vi "RichToFlatnixnet_grpc_ConnectTerminalsRequest.vi"(5 "OutputClusterType":T1, 11 "InputCluster":T4) -> (3 "OutputCluster":T1)   [LabVIEW 2025, in "grpc-xnet_client.lvlib"]
uses:
  grpc-xnet_client.lvlib
  nixnet_grpc_ConnectTerminalsRequest.ctl
  nixnet_grpc_ConnectTerminalsRequest_source_enum/nixnet_grpc_ConnectTerminalsRequest_source_enum.lvclass
  nixnet_grpc_ConnectTerminalsRequest_destination_enum/nixnet_grpc_ConnectTerminalsRequest_destination_enum.lvclass
  nidevice_grpc_Session.ctl
  nixnet_grpc_ConnectTerminalsRequest_Flat.ctl
  nidevice_grpc_Session_Flat.ctl
  nixnet_grpc_TerminalName.ctl
  nixnet_grpc_ConnectTerminalsRequest_source_enum/nixnet_grpc_ConnectTerminalsRequest_source_enum.lvclass/nixnet_grpc_ConnectTerminalsRequest_source_enum.ctl
  nixnet_grpc_ConnectTerminalsRequest_destination_enum/nixnet_grpc_ConnectTerminalsRequest_destination_enum.lvclass/nixnet_grpc_ConnectTerminalsRequest_destination_enum.ctl
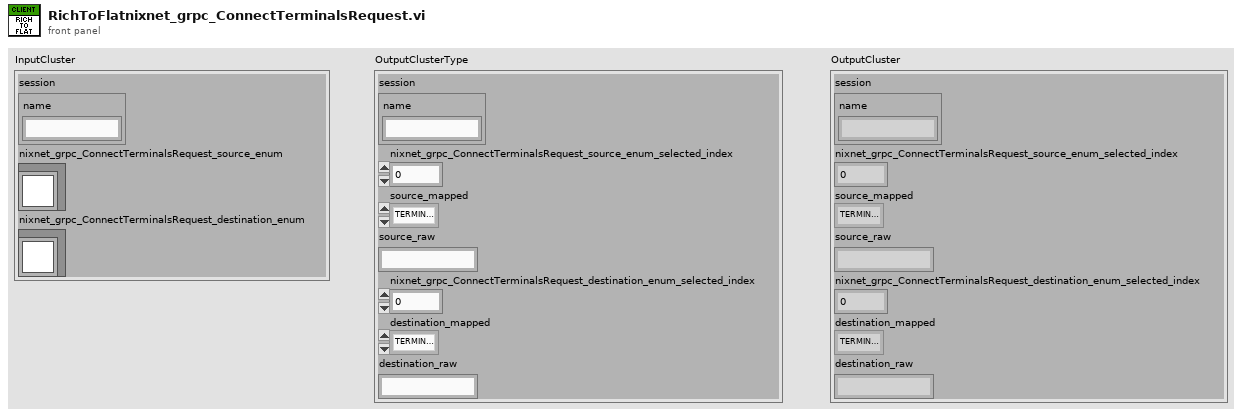
[diagram p1: front panel]
types:
  T1 = typedef "grpc-xnet_client.lvlib/nixnet_grpc_ConnectTerminalsRequest_Flat.ctl" = cluster{"session":T2, "nixnet_grpc_ConnectTerminalsRequest_source_enum_selected_index":i32, "source_mapped":T3, "source_raw":string, "nixnet_grpc_ConnectTerminalsRequest_destination_enum_selected_index":i32, "destination_mapped":T3, "destination_raw":string}
  T2 = typedef "grpc-xnet_client.lvlib/nidevice_grpc_Session_Flat.ctl" = cluster{"name":string}
  T3 = typedef "grpc-xnet_client.lvlib/nixnet_grpc_TerminalName.ctl" = enum32{"TERMINAL_NAME_UNSPECIFIED", "TERMINAL_NAME_PXI_TRIG_0", "TERMINAL_NAME_PXI_TRIG_1", "TERMINAL_NAME_PXI_TRIG_2", "TERMINAL_NAME_PXI_TRIG_3", "TERMINAL_NAME_PXI_TRIG_4", "TERMINAL_NAME_PXI_TRIG_5", "TERMINAL_NAME_PXI_TRIG_6", "TERMINAL_NAME_PXI_TRIG_7", "TERMINAL_NAME_FRONT_PANEL_0", "TERMINAL_NAME_FRONT_PANEL_1", "TERMINAL_NAME_PXI_STAR", "TERMINAL_NAME_PXI_CLK_10", "TERMINAL_NAME_10_MHZ_TIMEBASE", "TERMINAL_NAME_1_MHZ_TIMEBASE", "TERMINAL_NAME_MASTER_TIMEBASE", "TERMINAL_NAME_COMM_TRIGGER", "TERMINAL_NAME_START_TRIGGER", "TERMINAL_NAME_FLEX_RAY_START_CYCLE", "TERMINAL_NAME_FLEX_RAY_MACROTICK", "TERMINAL_NAME_LOG_TRIGGER", "TERMINAL_NAME_TIME_TRIGGER", "TERMINAL_NAME_NETWORK_TIME_PPS", "TERMINAL_NAME_NETWORK_TIME_1_MHZ"}
  T4 = typedef "grpc-xnet_client.lvlib/nixnet_grpc_ConnectTerminalsRequest.ctl" = cluster{"session":T5, "nixnet_grpc_ConnectTerminalsRequest_source_enum":refnum<class "nixnet_grpc_ConnectTerminalsRequest_source_enum.lvclass">, "nixnet_grpc_ConnectTerminalsRequest_destination_enum":refnum<class "nixnet_grpc_ConnectTerminalsRequest_destination_enum.lvclass">}
  T5 = typedef "grpc-xnet_client.lvlib/nidevice_grpc_Session.ctl" = cluster{"name":string}
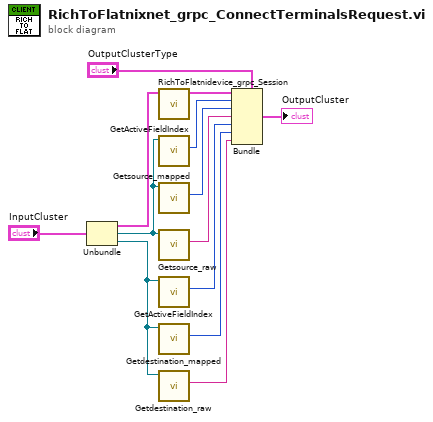
[diagram p0: block diagram]
diagram:
  n1 = Unbundle "Unbundle"("InputCluster") -> ("session"=w10:T5, "nixnet_grpc_ConnectTerminalsRequest_source_enum"=w8:refnum<class "nixnet_grpc_ConnectTerminalsRequest_source_enum.lvclass">, "nixnet_grpc_ConnectTerminalsRequest_destination_enum"=w4:refnum<class "nixnet_grpc_ConnectTerminalsRequest_destination_enum.lvclass">)
  n2 = call "RichToFlatnidevice_grpc_Session.vi"("InputCluster"=w10) -> ("OutputCluster"=w9:T2)  [unwired: 10 in]
  n3 = call "GetActiveFieldIndex.vi"("OneOfTemplate in"=w8) -> ("Active Field Index"=w7:i32)  [unwired: 8 in, 2 out]
  n4 = call "Getsource_mapped.vi"("OneOfTemplate in"=w8) -> ("Get_Val"=w6:T3)  [unwired: 8 in, 2 out]
  n5 = call "Getsource_raw.vi"("OneOfTemplate in"=w8) -> ("Get_Val"=w5:string)  [unwired: 8 in, 2 out]
  n6 = call "GetActiveFieldIndex.vi"("OneOfTemplate in"=w4) -> ("Active Field Index"=w3:i32)  [unwired: 8 in, 2 out]
  n7 = call "Getdestination_mapped.vi"("OneOfTemplate in"=w4) -> ("Get_Val"=w2:T3)  [unwired: 8 in, 2 out]
  n8 = call "Getdestination_raw.vi"("OneOfTemplate in"=w4) -> ("Get_Val"=w1:string)  [unwired: 8 in, 2 out]
  n9 = Bundle "Bundle"(cluster="OutputClusterType", "session"=w9, "nixnet_grpc_ConnectTerminalsRequest_source_enum_selected_index"=w7, "source_mapped"=w6, "source_raw"=w5, "nixnet_grpc_ConnectTerminalsRequest_destination_enum_selected_index"=w3, "destination_mapped"=w2, "destination_raw"=w1) -> (→"OutputCluster":T1)
